vi "Get CD Item Property Value.vi"(8 "error in (no error)":errorcluster, 10 "CD Item Ref in":u64, 11 "Boolean Parameter in":refnum<class "Boolean Parameter.lvclass">) -> (0 "error out":errorcluster, 3 "Boolean Parameter out":refnum<class "Boolean Parameter.lvclass">)   [LabVIEW 2016, in "CD Parameter Manager API.lvlib" / "Boolean Parameter.lvclass"]
uses:
  Boolean Parameter.lvclass
  <vilib>/NI VeriStand/Custom Device API/Custom Device API.lvlib
  <vilib>/NI VeriStand/Custom Device API/Get Item Property (Boolean).vi
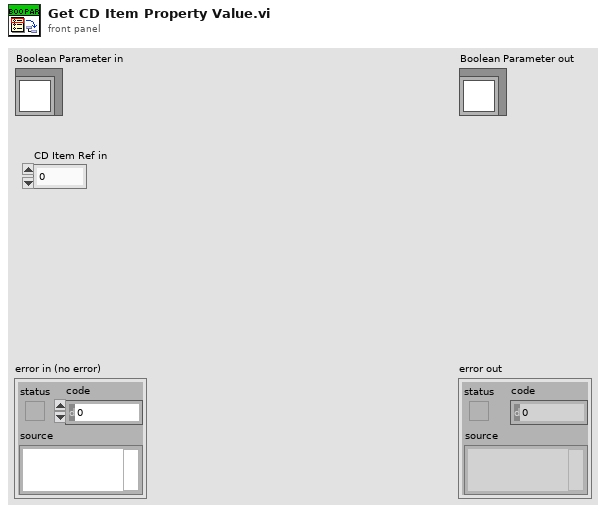
[diagram p1: front panel]
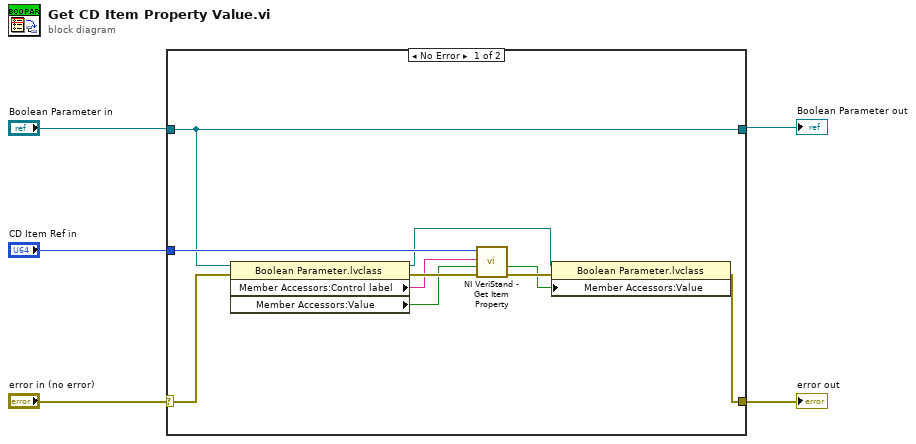
[diagram p0: block diagram]
diagram:
  n1 = case shown="No Error" "error in (no error)" {
    selector: "error in (no error)" -> [w14 w16]
    tunnel: [w8 w16] -> w3
    tunnel: "CD Item Ref in" -> [w15 _]
    tunnel: [w13 w17] -> w4
    tunnel: "Boolean Parameter in" -> [w13 w17]
    frame No Error {
      n2 = property class="Boolean Parameter.lvclass"(reference=w13, error in=w14) -> (reference out=w6:refnum<class "Boolean Parameter.lvclass">, error out=w12:errorcluster, "Member Accessors:Control label"=w11:string, "Member Accessors:Value"=w10:bool)
      n3 = call-poly <vilib>:"NI VeriStand - Get Item Property.vi"("error in (no error)"=w12, "Default Value"=w10, "Property Name"=w11, "Item Ref in"=w15) -> ("error out"=w9:errorcluster, "Value"=w7:bool)  [unwired: 4 in, 2 out]
      n4 = property class="Boolean Parameter.lvclass"(reference=w6, error in=w9, "Member Accessors:Value"=w7) -> (error out=w8:errorcluster)  [unwired: 1 out]
    }
    frame Error {
    }
  }
  "error out" <- w3
  "Boolean Parameter out" <- w4
